vi "grupowanie po promieniu.vi"(1 "Posortowana Tablica\nPo promieniu":dbl[][](array[numeric])) -> (0 "Grupy pkt \nO tych samych\nPromieniach":cluster{dbl[][]}[](array[cluster]))   [LabVIEW 2016]
doc: "To vi z posortowanej po promieniu tablicy pkt tworzy tablice clsutrów tablic o tym samym promieniu"
uses:
  <vilib>/express/express arith-compare/Formula/XNode/ExpressFormulaBlockNode.xnode
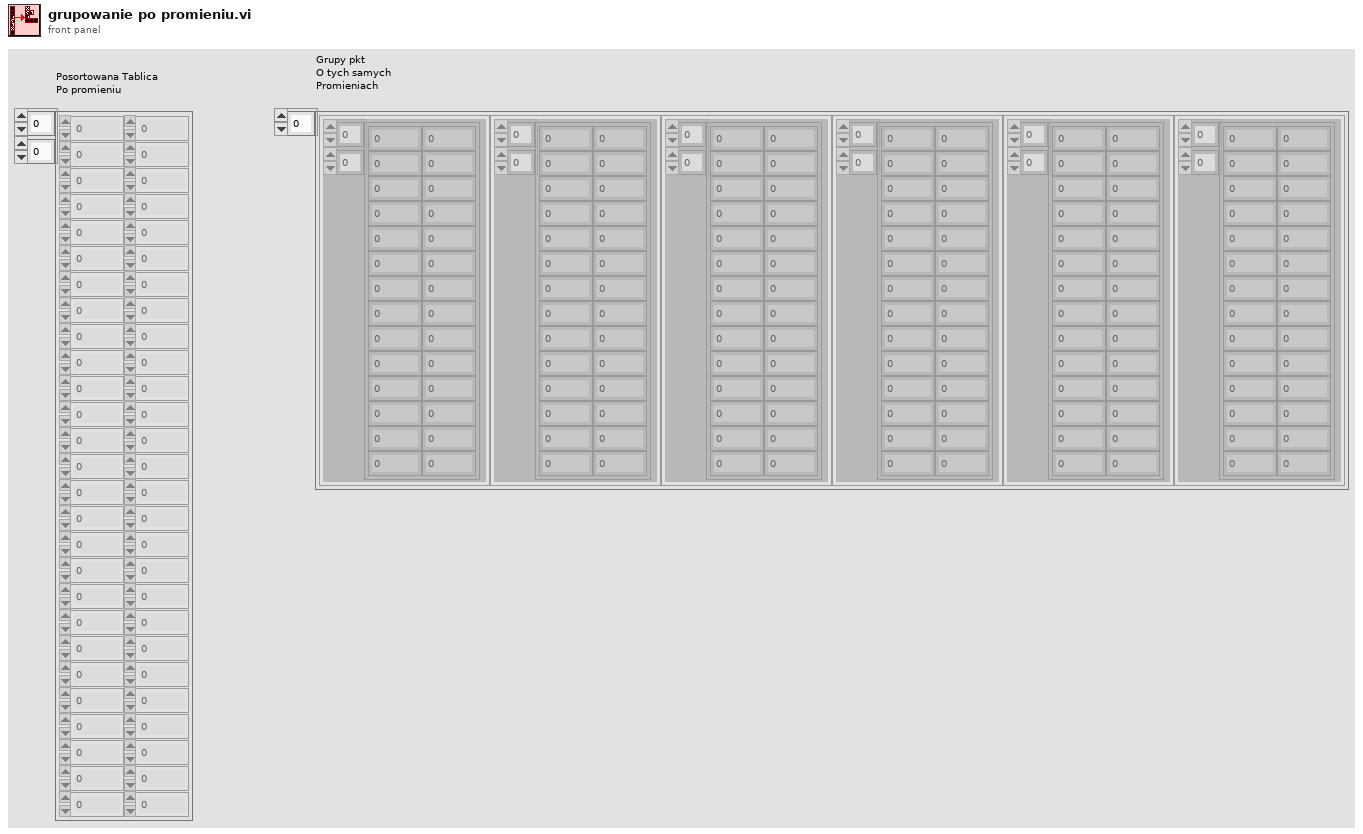
[diagram p1: front panel]
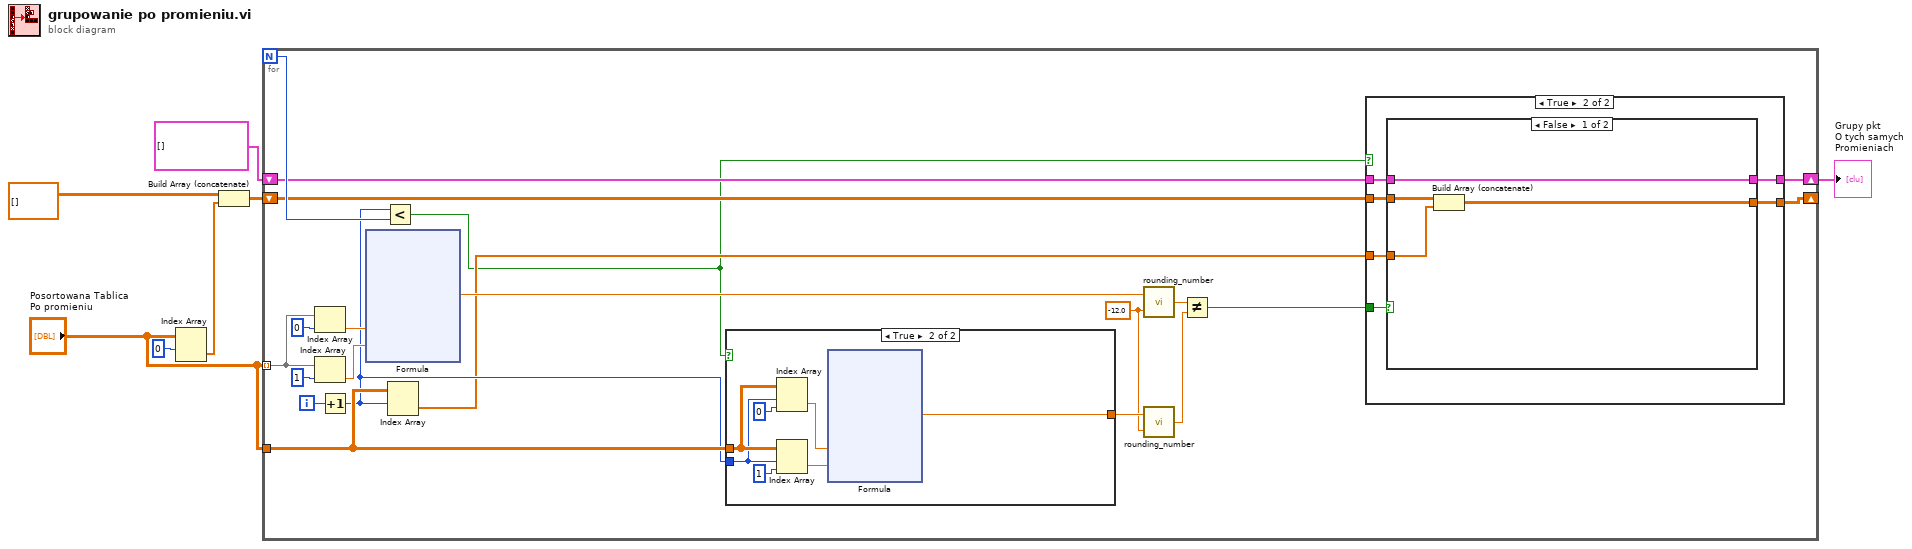
[diagram p0: block diagram]
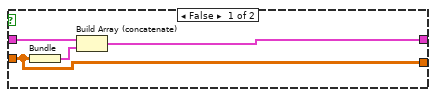
[diagram p2: hidden frame]
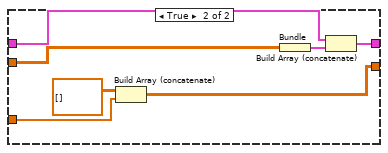
[diagram p3: hidden frame]
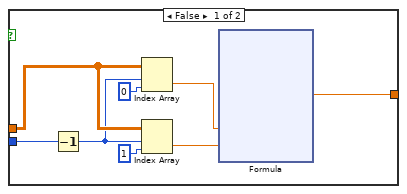
[diagram p4: hidden frame]
diagram:
  n1 = Index Array(array="Posortowana Tablica\nPo promieniu", index (row)=0) -> (element=w3:dbl[])  [unwired: 1 in]
  n2 = Build Array (concatenate)(dbl[][] [], w3) -> (w6:dbl[][])
  n3 = for {
    N -> [w25]
    tunnel: "Posortowana Tablica\nPo promieniu" -> [w24] mode=indexing
    tunnel: "Posortowana Tablica\nPo promieniu" -> [w14]
    shift-right: [w11] -> _
    shift-left: w6 -> [w15]
    shift-right: [w9] -> w1
    shift-left: cluster{dbl[][]}[] [] -> [w10]
    i -> [w26]
    w19 = -12.0 ("Power of ten")
    n4 = Index Array(array=w24, index=0) -> (element=w23:dbl)
    n5 = Index Array(array=w24, index=1) -> (element=w22:dbl)
    n6 = Increment(x=w26) -> (x+1=w13:i32)
    n7 = xnode "Formula"("x"=w23, "y"=w22) -> ("Result"=w21:dbl)  [unwired: 1 in, 1 out]
    n8 = Less?(x=w13, y=w25) -> (x < y?=w8:bool)
    n9 = Index Array(array=w14, index (row)=w13) -> (element=w12:dbl[])  [unwired: 1 in]
    n10 = case shown="True" w8 {
      tunnel: w13 -> [w67 w83]
      tunnel: w14 -> [w62 w84]
      tunnel: [w60 w78] -> w20
      frame False {
        n11 = Decrement(x=w67) -> (x-1=w61:i32)
        n12 = Index Array(array=w62, index (row)=w61, index (col)=0 ("disabled index (col)")) -> (element=w64:dbl)
        n13 = Index Array(array=w62, index (row)=w61, index (col)=1 ("disabled index (col)")) -> (element=w63:dbl)
        n14 = xnode "Formula"("x"=w64, "y"=w63) -> ("Result"=w60:dbl)  [unwired: 1 in, 1 out]
      }
      frame True {
        n15 = Index Array(array=w84, index (row)=w83, index (col)=0 ("disabled index (col)")) -> (element=w80:dbl)
        n16 = Index Array(array=w84, index (row)=w83, index (col)=1 ("disabled index (col)")) -> (element=w79:dbl)
        n17 = xnode "Formula"("x"=w80, "y"=w79) -> ("Result"=w78:dbl)  [unwired: 1 in, 1 out]
      }
    }
    n18 = call "rounding_number.vi"("Power of ten"=w19, "Number to round"=w21) -> ("Rounded number"=w18:dbl)
    n19 = call "rounding_number.vi"("Power of ten"=w19, "Number to round"=w20) -> ("Rounded number"=w17:dbl)
    n20 = Not Equal?(x=w18, y=w17) -> (x != y?=w16:bool)
    n21 = case shown="True" w8 {
      tunnel: w16 -> [_ w38]
      tunnel: w15 -> [w29 w37]
      tunnel: w12 -> [_ w36]
      tunnel: [w29 w35] -> w11
      tunnel: w10 -> [w31 w34]
      tunnel: [w30 w33] -> w9
      frame False {
        n22 = Bundle(w29) -> (w32:cluster{dbl[][]})  [unwired: 1 in]
        n23 = Build Array (concatenate)(w31, w32) -> (w30:cluster{dbl[][]}[])
      }
      frame True {
        n24 = case shown="False" w38 {
          tunnel: w37 -> [w42 w46]
          tunnel: w36 -> [w41 w48]
          tunnel: [w40 w47] -> w35
          tunnel: w34 -> [w39 w44]
          tunnel: [w39 w43] -> w33
          frame False {
            n25 = Build Array (concatenate)(w42, w41) -> (w40:dbl[][])
          }
          frame True {
            n26 = Build Array (concatenate)(dbl[][] [], w48) -> (w47:dbl[][])
            n27 = Bundle(w46) -> (w45:cluster{dbl[][]})  [unwired: 1 in]
            n28 = Build Array (concatenate)(w44, w45) -> (w43:cluster{dbl[][]}[])
          }
        }
      }
    }
  }
  "Grupy pkt \nO tych samych\nPromieniach" <- w1
